vi "open chromatogram.vi"() -> (2 "GC record":T1 {"delta x" format="%.4f"; "chromatogram 1" format="%.2f"})   [LabVIEW 2012]
uses:
  GC record.ctl
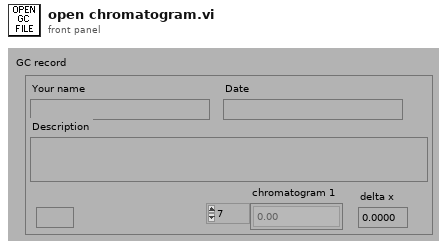
[diagram p1: front panel]
types:
  T1 = typedef "GC record.ctl" = cluster{"chromatogram 1":dbl[], "Your name":string, "Description":string, "Date":string, "delta x":dbl, "Det in use":string}
  T2 = enum16{"open", "open or create", "create or replace", "create", "open (read only)"}
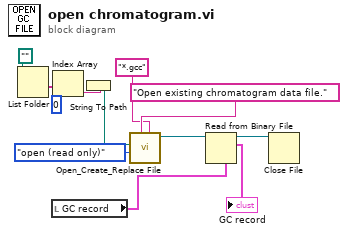
[diagram p0: block diagram]
diagram:
  n1 = List Folder(path=path "") -> (folder names=w7:string[])  [unwired: 3 in, 3 out]
  n2 = local read "GC record"() -> (w2:T1)
  n3 = Index Array(array=w7, index=0) -> (element=w9:string)
  n4 = String To Path(string=w9) -> (path=w6:path)
  n5 = call <vilib>:"Open_Create_Replace File.vi"("pattern"="*.gcc", "prompt"="Open existing chromatogram data file.", "function (open:0)"=T2."open (read only)", "start path  (Not A Path)"=w6) -> ("refnum"=w3:refnum<file>)  [unwired: 4 in, 3 out]
  n6 = Read from Binary File(5:w2, 11:w3) -> (2:→"GC record":T1, 3:w12:refnum<file>)  [unwired: 4 in, 2 out]
  n7 = Close File(refnum=w12) -> ()  [unwired: 1 in, 2 out]
